vi "Fresnel Integrals.vi"(3 "x":dbl format="%.2f") -> (0 "S(x)":dbl format="%.2f", 1 "C(x)":dbl format="%.2f")   [LabVIEW 2017, in "NI_Gmath.lvlib"]
doc: "Computes the Fresnel cosine and sine integral functions."
uses:
  <vilib>/gmath/NI_Gmath.lvlib
  <resource>/lvanlys.dll
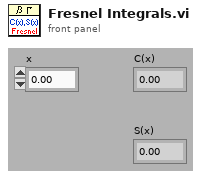
[diagram p1: front panel]
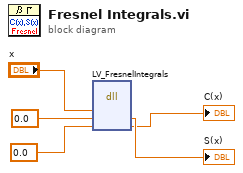
[diagram p0: block diagram]
diagram:
  n1 = dll-call lib="e:/builds/penguin/labview/branches/2017/dev/dist/resource/lvanlys.*" fn="LV_FresnelIntegrals"("x"="x", "fSinI"=0.0, "fCosI"=0.0) -> ("fSinI"=→"S(x)":dbl, "fCosI"=→"C(x)":dbl)  [unwired: 5 in, 2 out]
